vi "Encode Frame ID.vi"(9 "ISO FD Type":T1=enum."CAN 2.0", 10 "Extended ID":bool, 11 "Frame ID in":u32=12) -> (3 "Frame ID out":u32=12)   [LabVIEW 2021, in "CAN_Logic.lvclass"]
uses:
  CAN_Logic.lvclass
  typedef/ISO FD Frame Type.ctl
  CAN_Logic.lvclass/CAN_Logic.ctl
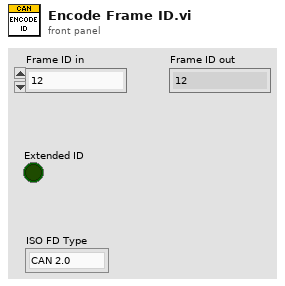
[diagram p1: front panel]
types:
  T1 = typedef "CAN_Logic.lvclass/ISO FD Frame Type.ctl" = enum16{"Not Specified", "CAN 2.0", "FD", "FD+BRS"}
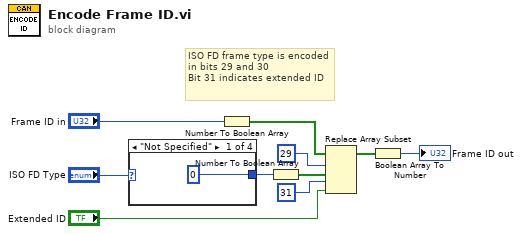
[diagram p0: block diagram]
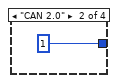
[diagram p2: hidden frame]
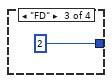
[diagram p3: hidden frame]
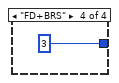
[diagram p4: hidden frame]
diagram:
  # "ISO FD frame type is encoded in bits 29 and 30\nBit 31 indicates extended ID"
  n1 = case shown="\"Not Specified\"" "ISO FD Type" {
    tunnel: [u8 0 u8 1 u8 2 u8 3] -> w8
    frame "Not Specified" {
    }
    frame "CAN 2.0" {
    }
    frame "FD" {
    }
    frame "FD+BRS" {
    }
  }
  n2 = Number To Boolean Array(number="Frame ID in") -> (Boolean array=w7:bool[])
  n3 = Number To Boolean Array(number=w8) -> (Boolean array=w1:bool[])
  n4 = Replace Array Subset(array=w7, new element #1=w1, index #1=29 ("index"), new element #2="Extended ID", index #2=31 ("index")) -> (w3:bool[])
  n5 = Boolean Array To Number(Boolean array=w3) -> (number=→"Frame ID out":u32)
